vi "CreateArrayOfValues.vi"(1 "error out":errorcluster, 2 "Image Out":T1) -> (0 "Array":dbl[](array[numeric]))   [LabVIEW 2009]
uses:
  <vilib>/vision/Image Controls.llb/IMAQ Image.ctl
  <vilib>/vision/NI_Vision_Development_Module.lvlib
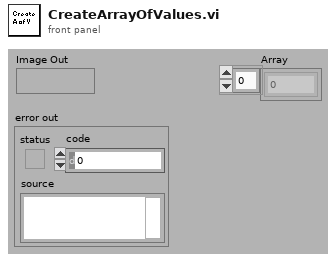
[diagram p1: front panel]
types:
  T1 = typedef "IMAQ Image.ctl" = refnum<image>
  T2 = cluster{"Red (or Hue) value":u8, "Green (or Sat) value":u8, "Blue (or Light or Val) value":u8}[][]
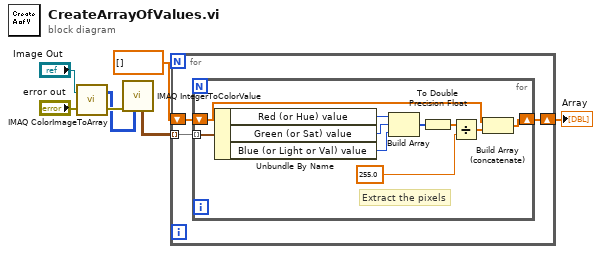
[diagram p0: block diagram]
diagram:
  n1 = call "IMAQ ColorImageToArray"("Image"="Image Out", "error in (no error)"="error out") -> ("Image Pixels (U32)"=w3:u32[][], "error out"=w4:errorcluster)  [unwired: 2 in, 1 out]
  n2 = call "IMAQ IntegerToColorValue"("error in (no error)"=w4, "2D U32 array"=w3) -> ("2D Color value array"=w5:T2)  [unwired: 3 in, 3 out]
  n3 = for {
    tunnel: w5 -> [w10] mode=indexing
    shift-right: [w9] -> w7
    shift-left: dbl[] [] -> [w8]
    n4 = for {
      tunnel: w10 -> [w20] mode=indexing
      shift-right: [w16] -> w9
      shift-left: w8 -> [w15]
      # "Extract the pixels"
      n5 = Unbundle By Name(w20) -> ("Red (or Hue) value"=w19:u8, "Green (or Sat) value"=w18:u8, "Blue (or Light or Val) value"=w17:u8)
      n6 = Build Array(w19, w18, w17) -> (w14:u8[])
      n7 = To Double Precision Float(number=w14) -> (double precision float=w13:dbl[])
      n8 = Divide(x=w13, y=255.0 ("Blue (or Light or Val) value")) -> (x/y=w12:dbl[])
      n9 = Build Array (concatenate)(w15, w12) -> (w16:dbl[])
    }
  }
  "Array" <- w7
